vi "NF WF1973_74 TRIG Tim.vi"(4 "Set(Sweep)":bool, 5 "Units(S)":u16(ring)=2 items=["S", "Milli(m)", "Micro(u)"], 6 "Read(F)":bool, 7 "Period(1)":dbl=1.0 min=0.0001 max=10000.0 step=1e-05 format="%.7f", 8 "error in (no error)":errorcluster caption="Error IN", 9 "Trigger Period(Input)":u16(ring) items=["Input", "Minimum", "Maximum"], 10 "Ch(Ch1)":bool, 11 "VISAsession":refnum<visa-resource-name>) -> (0 "error out":errorcluster caption="Error OUT", 2 "Query Trigger Period":dbl format="%.7f", 3 "CopyVISAsession":refnum<visa-resource-name>)   [LabVIEW 2010]
panel:
  # "Choose\nInput"
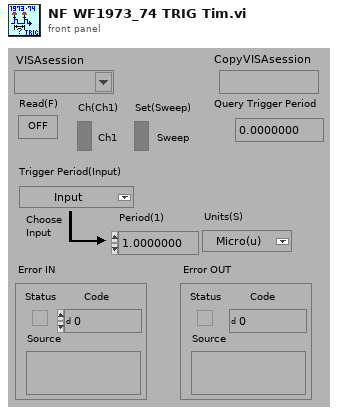
[diagram p1: front panel]
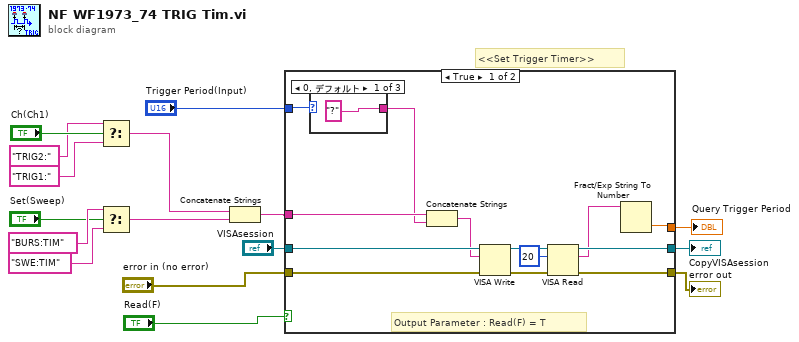
[diagram p0: block diagram]
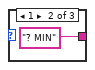
[diagram p2: hidden frame]
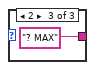
[diagram p3: hidden frame]
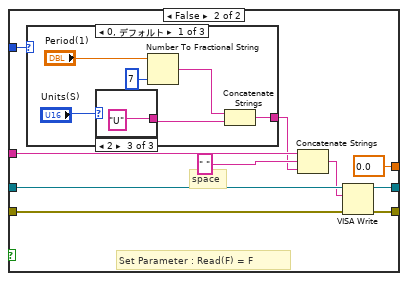
[diagram p4: hidden frame]
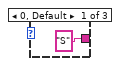
[diagram p5: hidden frame]
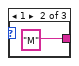
[diagram p6: hidden frame]
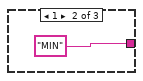
[diagram p7: hidden frame]
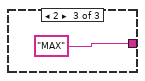
[diagram p8: hidden frame]
diagram:
  # "<<Set Trigger Timer>>"
  n1 = Select(t="TRIG2:" ("文字列"), s="Ch(Ch1)", f="TRIG1:" ("文字列")) -> (s? t:f=w2:string)
  n2 = Select(t="BURS:TIM", s="Set(Sweep)", f="SWE:TIM") -> (s? t:f=w1:string)
  n3 = Concatenate Strings(w2, w1) -> (w3:string)
  n4 = case shown="TRUE" "Read(F)" {
    tunnel: "VISAsession" -> [w29 w42]
    tunnel: [w26 w40] -> w15
    tunnel: [w25 w41] -> w14
    tunnel: "error in (no error)" -> [w24 w37]
    tunnel: w3 -> [w22 w38]
    tunnel: [w21 0.0] -> w11
    tunnel: "Trigger Period(Input)" -> [w19 w36]
    frame True {
      # "Output Parameter : Read(F) = T"
      n5 = case shown="0, デフォルト" w19 {
        tunnel: ["?" ("形式文字列") "? MIN" ("形式文字列") "? MAX" ("形式文字列")] -> w18
        frame 0, Default {
        }
        frame 1 {
        }
        frame 2 {
        }
      }
      n6 = Concatenate Strings(w22, w18) -> (w17:string)
      n7 = VISA Write(VISA resource name=w29, write buffer=w17, error in (no error)=w24) -> (VISA resource name out=w27:refnum<visa-resource-name>, error out=w28:errorcluster)  [unwired: 1 out]
      n8 = VISA Read(VISA resource name=w27, byte count=u32 20 ("バイトカウント（0）"), error in (no error)=w28) -> (VISA resource name out=w26:refnum<visa-resource-name>, read buffer=w20:string, error out=w25:errorcluster)  [unwired: 1 out]
      n9 = Fract/Exp String To Number(string=w20) -> (number=w21:dbl)  [unwired: 3 in, 1 out]
    }
    frame False {
      # "space"
      # "Set Parameter : Read(F) = F"
      n10 = case shown="0, デフォルト" w36 {
        tunnel: [w47 "MIN" ("文字列") "MAX" ("文字列")] -> w35
        frame 0, Default {
          n11 = case shown="2" "Units(S)" {
            tunnel: ["S" "M" "U"] -> w43
            frame 0, Default {
            }
            frame 1 {
            }
            frame 2 {
            }
          }
          n12 = Number To Fractional String(number="Period(1)", precision (6)=i16 7 ("精度 (6)")) -> (F-format string=w44:string)  [unwired: 2 in]
          n13 = Concatenate Strings(w44, w43) -> (w47:string)
        }
        frame 1 {
        }
        frame 2 {
        }
      }
      n14 = Concatenate Strings(w38, " ", w35) -> (w33:string)
      n15 = VISA Write(VISA resource name=w42, write buffer=w33, error in (no error)=w37) -> (VISA resource name out=w40:refnum<visa-resource-name>, error out=w41:errorcluster)  [unwired: 1 out]
    }
  }
  "error out" <- w14
  "CopyVISAsession" <- w15
  "Query Trigger Period" <- w11
